vi "XY-Data to Dictionary (single).vi"(8 "error in (no error)":errorcluster, 10 "Name":string, 11 "XY-data in":cluster{"X-array":dbl[], "Y-array":dbl[]} {"Y-array" format="%.2p"; "X-array" format="%.2p"}) -> (0 "error out":errorcluster, 3 "Data (Dictionary)":T1[](array[typedef]))   [LabVIEW 2016, in "Data.lvclass"]
uses:
  Data.lvclass
  Typedefs/Dictionary--cluster.ctl
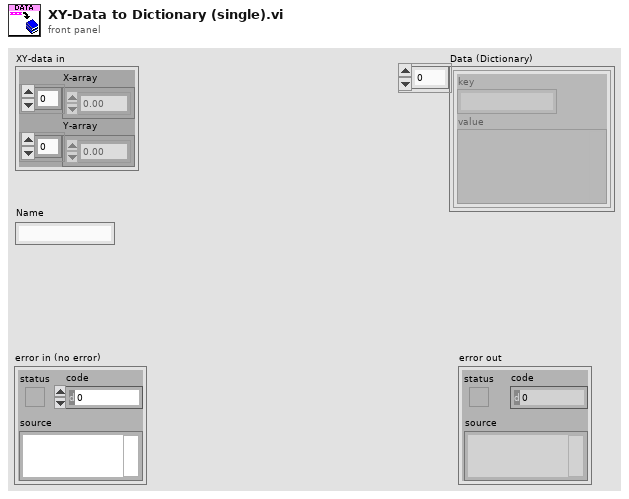
[diagram p1: front panel]
types:
  T1 = typedef "Data.lvclass/Dictionary--cluster.ctl" = cluster{"key":string, "value":variant}
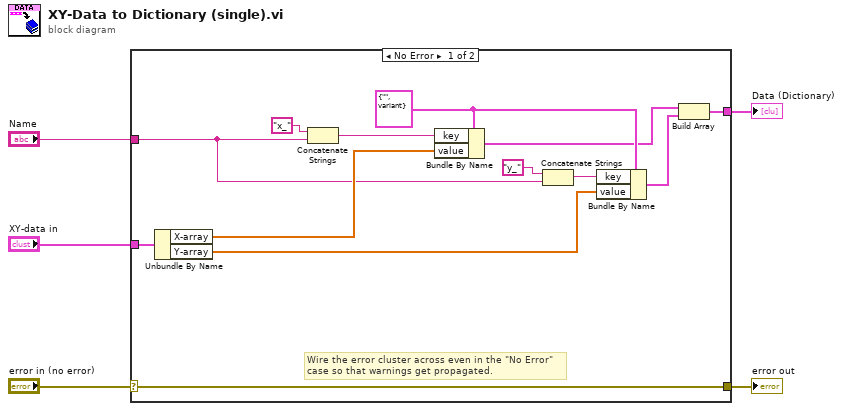
[diagram p0: block diagram]
diagram:
  n1 = case shown="No Error" "error in (no error)" {
    selector: "error in (no error)" -> [w18 w19]
    tunnel: [w18 w19] -> w4
    tunnel: "XY-data in" -> [w17 _]
    tunnel: [w8 _] -> w2
    tunnel: "Name" -> [w11 _]
    frame No Error {
      w9 = T1 {"key"="", "value"=variant} ("key-value")
      # "Wire the error cluster across even in the \"No Error\"\ncase so that warnings get propagated."
      n2 = Unbundle By Name(w17) -> ("X-array"=w14:dbl[], "Y-array"=w10:dbl[])
      n3 = Concatenate Strings("x_" ("string"), w11) -> (w15:string)
      n4 = Bundle By Name(cluster=w9, "key"=w15, "value"=w14) -> (w7:T1)
      n5 = Concatenate Strings("y_" ("string"), w11) -> (w12:string)
      n6 = Bundle By Name(cluster=w9, "key"=w12, "value"=w10) -> (w6:T1)
      n7 = Build Array(w7, w6) -> (w8:T1[])
    }
    frame Error {
    }
  }
  "error out" <- w4
  "Data (Dictionary)" <- w2
